vi "Fill in Off Time.vi"(10 "Start Time":string, 11 "Data IN":string[][](array[string])) -> (2 "Sample Rate":dbl, 3 "Data OUT":sgl[][](array[numeric]))   [LabVIEW 2023]
panel:
  out "Waveform Graph":sgl[][](graph)
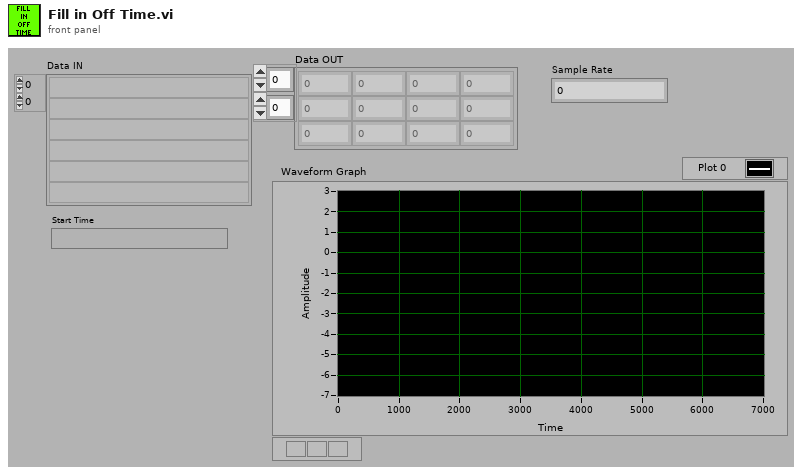
[diagram p1: front panel]
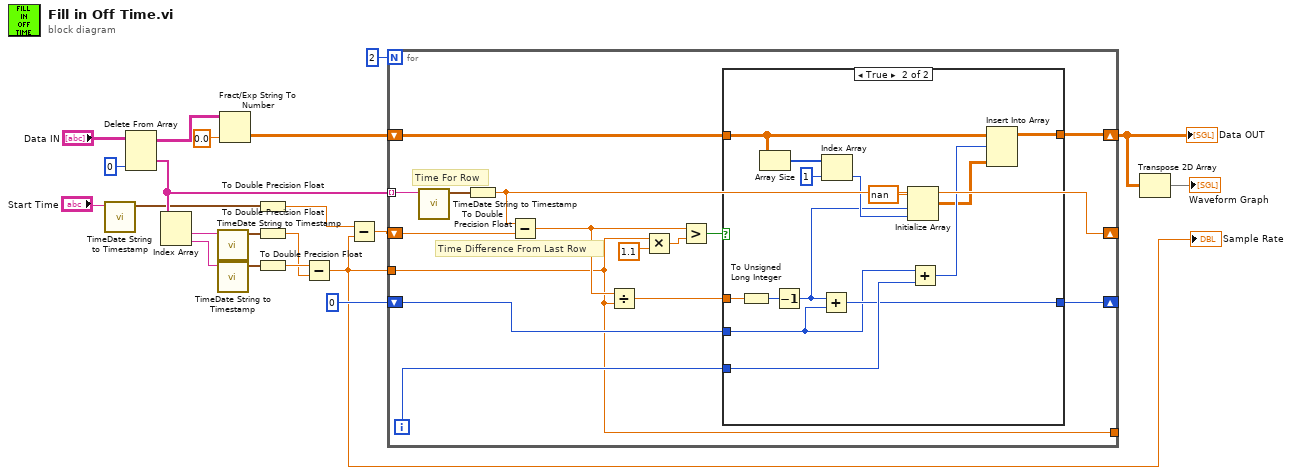
[diagram p0: block diagram]
diagram:
  n1 = call "TimeDate String to Timestamp.vi"("Time/Date String"="Start Time") -> ("Timestamp"=w7:timestamp)  [unwired: 10 in]
  n2 = Delete From Array(array="Data IN", index (col)=0 ("disabled index (col)")) -> (deleted portion=w17:string[], array with subset deleted=w18:string[][])  [unwired: 2 in]
  n3 = Index Array(array=w17) -> (element #1=w16:string, element #2=w15:string)  [unwired: 2 in]
  n4 = call "TimeDate String to Timestamp.vi"("Time/Date String"=w16) -> ("Timestamp"=w14:timestamp)  [unwired: 10 in]
  n5 = call "TimeDate String to Timestamp.vi"("Time/Date String"=w15) -> ("Timestamp"=w13:timestamp)  [unwired: 10 in]
  n6 = Fract/Exp String To Number(string=w18, default (0 dbl)=sgl 0.0 ("default (0 DBL)")) -> (number=w10:sgl[][])  [unwired: 2 in, 1 out]
  n7 = To Double Precision Float(number=w7) -> (double precision float=w4:dbl)
  n8 = To Double Precision Float(number=w14) -> (double precision float=w5:dbl)
  n9 = To Double Precision Float(number=w13) -> (double precision float=w12:dbl)
  n10 = Subtract(x=w12, y=w5) -> (x-y=w3:dbl)
  "Sample Rate" <- w3
  n11 = Subtract(x=w4, y=w3) -> (x-y=w2:dbl)
  n12 = for {
    N: 2 -> [_]
    tunnel: w17 -> [w36] mode=indexing
    tunnel: w3 -> [w22]
    shift-right: [w34] -> _
    shift-left: w2 -> [w23]
    shift-right: [w30] -> _
    shift-left: u32 0 -> [w29]
    shift-right: [w27] -> w6
    shift-left: w10 -> [w28]
    tunnel: [w22] -> _
    i -> [w24]
    # "Time Difference From Last Row"
    # "Time For Row"
    n13 = call "TimeDate String to Timestamp.vi"("Time/Date String"=w36) -> ("Timestamp"=w35:timestamp)  [unwired: 10 in]
    n14 = To Double Precision Float(number=w35) -> (double precision float=w34:dbl)
    n15 = Subtract(x=w34, y=w23) -> (x-y=w33:dbl)
    n16 = Divide(x=w33, y=w22) -> (x/y=w31:dbl)
    n17 = Multiply(x=w22, y=1.1) -> (x*y=w26:dbl)
    n18 = Greater?(x=w33, y=w26) -> (0:w32:bool)
    n19 = case shown="True" w32 {
      tunnel: w31 -> [_ w52]
      tunnel: [w38 w44] -> w30
      tunnel: w29 -> [w38 w41]
      tunnel: w28 -> [w37 w50]
      tunnel: [w37 w51] -> w27
      tunnel: w24 -> [_ w45]
      frame False {
      }
      frame True {
        n20 = To Unsigned Long Integer(number=w52) -> (unsigned 32bit integer=w40:u32)
        n21 = Array Size(array=w50) -> (size(s)=w49:i32[])
        n22 = Decrement(x=w40) -> (x-1=w39:u32)
        n23 = Add(x=w39, y=w41) -> (x+y=w44:u32)
        n24 = Index Array(array=w49, index=1) -> (element=w46:i32)
        n25 = Initialize Array(nan ("default (0 DBL)"), w39, w46) -> (w42:dbl[][])
        n26 = Add(x=w41, y=w45) -> (x+y=w43:u32)
        n27 = Insert Into Array(array=w50, index (row)=w43, new element=w42) -> (w51:sgl[][])  [unwired: 1 in]
      }
    }
  }
  "Data OUT" <- w6
  n28 = Transpose 2D Array(2D array=w6) -> (transposed array=→"Waveform Graph":sgl[][])
